vi "Obtain Transfer Group.vi"(8 "error in (no error)":errorcluster, 10 "command parameters":T1, 11 "Transceiver Thread in":refnum<class "Plugin Thread.lvclass">) -> (0 "error out":errorcluster, 2 "Transfer Group":refnum<class "Transfer Group.lvclass">, 3 "Transceiver Thread out":refnum<class "Plugin Thread.lvclass">)   [LabVIEW 2017, in "DSF Core.lvlib" / "Plugin Thread.lvclass"]
uses:
  Thread/Plugin/Plugin Thread.lvclass
  Interface/Plugin/Command Parameters.ctl
  Transfer Group/Transfer Group.lvclass
  Interface/Plugin/Plugin Interface.lvclass
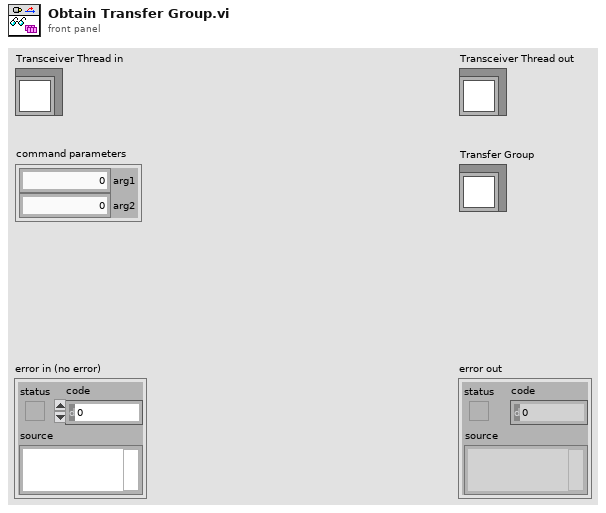
[diagram p1: front panel]
types:
  T1 = typedef "DSF Core.lvlib/Plugin Interface.lvclass/Command Parameters.ctl" = cluster{"arg1":u64, "arg2":u64}
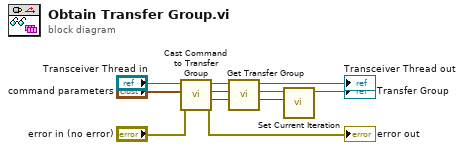
[diagram p0: block diagram]
diagram:
  n1 = call "Cast Command to Transfer Group.vi"("error in (no error)"="error in (no error)", "command parameters"="command parameters", "Plugin Thread in"="Transceiver Thread in") -> ("error out"=→"error out":errorcluster, "Transfer Group iteration"=w8:u64, "Transfer Group id"=w5:i32, "Plugin Thread out"=w6:refnum<class "Plugin Thread.lvclass">)  [unwired: 5 in]
  n2 = call "Get Transfer Group.vi"("index"=w5, "Transceiver Thread in"=w6) -> ("Transfer Group"=w3:refnum<class "Transfer Group.lvclass">, "Transceiver Thread out"=→"Transceiver Thread out":refnum<class "Plugin Thread.lvclass">)  [unwired: 8 in]
  n3 = call "Set Current Iteration.vi"("iteration"=w8, "Transfer Group in"=w3) -> ("Transfer Group out"=→"Transfer Group":refnum<class "Transfer Group.lvclass">)  [unwired: 9 in]
